vi "Transfer.Get Channel Blocks.vi"(11 "Transfer in":refnum<class "Transfer.lvclass">) -> (2 "channel blocks":T1[](array[typedef]) {"buffer offset" format="%d bytes"}, 3 "Transfer out":refnum<class "Transfer.lvclass">)   [LabVIEW 2017, in "DSF.Engine.lvlib" / "Transfer.lvclass"]
uses:
  Transfer.lvclass
  Shared/Typedefs/DSF Runtime Channel Block.ctl
  DSF Configuration API/1.0.0/Public/Controls/DSF Data Type.ctl
  Transfer.lvclass/Transfer.ctl
  DSF.Engine.lvlib
  DSF Configuration API/1.0.0/DSF Configuration API.lvlib
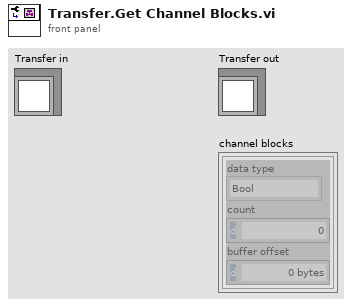
[diagram p1: front panel]
types:
  T1 = typedef "DSF.Engine.lvlib/DSF Runtime Channel Block.ctl" = cluster{"data type":T2, "count":u64, "buffer offset":u64}
  T2 = typedef "DSF Configuration API.lvlib/DSF Data Type.ctl" = enum8{"Bool", "SGL", "DBL", "I8", "I16", "I32", "I64", "U8", "U16", "U32", "U64"}
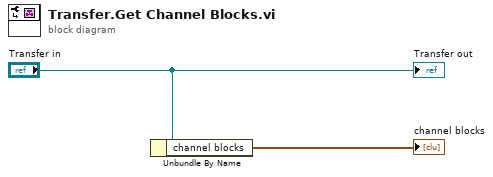
[diagram p0: block diagram]
diagram:
  n1 = Unbundle By Name("Transfer in") -> ("channel blocks"=→"channel blocks":T1[])
  "Transfer out" <- "Transfer in"
